vi "PPL_ActionVIOnCompile.vi"(8 "error in (no error)":errorcluster, 11 "Device Item Ref in":T1 format="%.0x") -> (0 "error out":errorcluster)   [LabVIEW 2019]
uses:
  <vilib>/NI VeriStand/Custom Device API/Custom Device Item Ref.ctl
  <vilib>/NI VeriStand/Custom Device Tools/Custom Device Utility Library/NI VeriStand - Search for Item by Name.vi
  <vilib>/NI VeriStand/Custom Device API/Set Item Property (Variant).vi
  <vilib>/NI VeriStand/Custom Device Tools/Custom Device Utility Library/Custom Device Utility Library.lvlib
  <vilib>/NI VeriStand/Custom Device API/Custom Device API.lvlib
  <vilib>/NI/NIVS Inline Async API/_Data Access System Explorer/Data Access System Explorer.lvlib
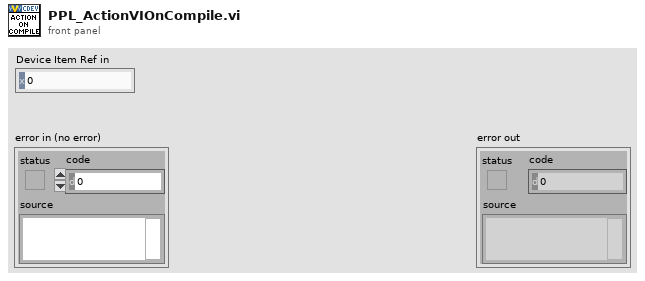
[diagram p1: front panel]
types:
  T1 = typedef "Custom Device API.lvlib/Custom Device Item Ref.ctl" = u64
  T2 = cluster{"Name":string, "Type":enum16{"Output/Write", "Input/Read", "Input/ReadWrite"}, "VS Refs":T1[]}
  T3 = enum16{"Output/Write", "Input/Read", "Input/ReadWrite"}
  T4 = typedef "Custom Device API.lvlib/Custom Device Item Info.ctl" = cluster{"Name":string, "Is Channel":bool, "GUID":string, "Is Waveform":bool}
  T5 = cluster{"Name":string, "Type":enum16{"Output/Write", "Input/Read", "Input/ReadWrite"}, "VS Refs":T1[]}[]
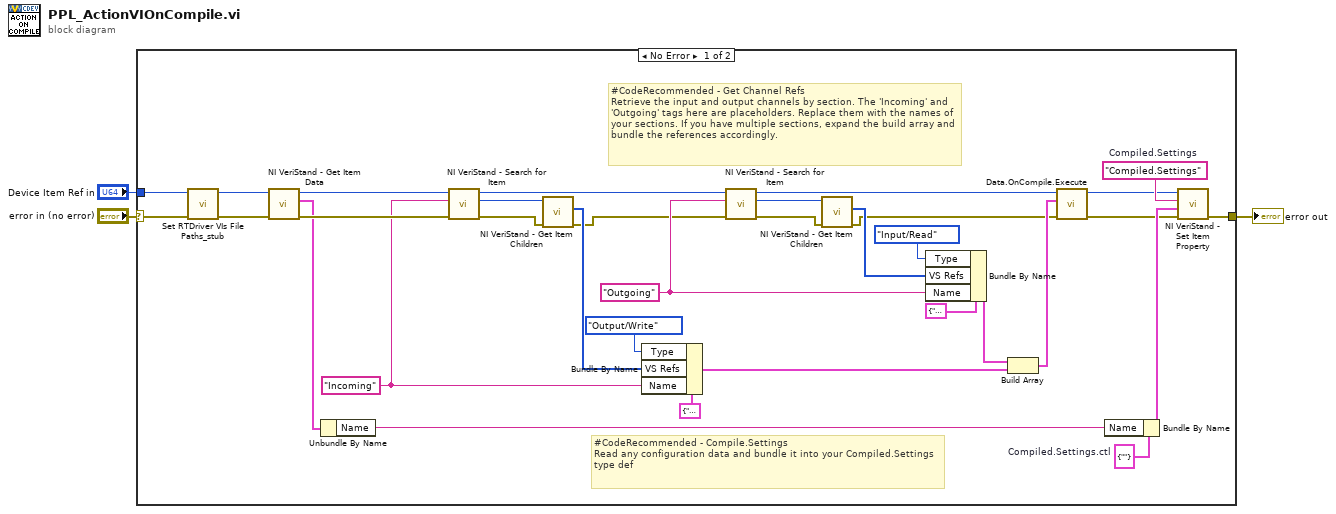
[diagram p0: block diagram]
diagram:
  n1 = case shown="No Error" "error in (no error)" {
    selector: "error in (no error)" -> [w4 w37]
    tunnel: [w30 w37] -> w2
    tunnel: "Device Item Ref in" -> [w7 _]
    frame No Error {
      w8 = cluster{"Name":string} {"Name"=""}  # Compiled.Settings.ctl
      w23 = "Outgoing" ("Item Name")
      w25 = "Incoming" ("Item Name")
      w32 = "Compiled.Settings"  # Compiled.Settings
      # "#CodeRecommended - Get Channel Refs\nRetrieve the input and output channels by section. The 'Incoming' and 'Outgoing' tags here are placeholders. Replace them with the names of your sections. If you have multiple sections, expand the build array and bundle the references accordingly."
      # "#CodeRecommended - Compile.Settings\nRead any configuration data and bundle it into your Compiled.Settings type def"
      n2 = call "Set RTDriver VIs File Paths_stub.vi"("error in (no error)"=w4, "Item Ref in"=w7) -> ("error out"=w5:errorcluster, "Item Ref out"=w6:T1)  [unwired: 8 in]
      n3 = call <vilib>:"NI VeriStand - Get Item Data.vi"("error in (no error)"=w5, "Item Ref in"=w6) -> ("error out"=w28:errorcluster, "Item Info"=w27:T4, "Item Ref out"=w29:T1)  [unwired: 6 in, 1 out]
      n4 = Unbundle By Name(w27) -> ("Name"=w26:string)
      n5 = call-poly <vilib>:"NI VeriStand - Search for Item.vi"("error in"=w28, "Item Name"=w25, "Section Ref in"=w29) -> ("error out"=w36:errorcluster, "Item Ref"=w35:T1, "Section Ref out"=w12:T1)  [unwired: 5 in, 1 out]
      n6 = call <vilib>:"NI VeriStand - Get Item Children.vi"("error in (no error)"=w36, "Item Ref in"=w35) -> ("error out"=w11:errorcluster, "Child Refs"=w24:T1[])  [unwired: 6 in, 2 out]
      n7 = Bundle By Name(cluster=T2 {"Name"="", "Type"=enum."Output/Write", "VS Refs"=[]} ("Group"), "Type"=T3."Output/Write", "VS Refs"=w24, "Name"=w25) -> (w15:T2)
      n8 = call-poly <vilib>:"NI VeriStand - Search for Item.vi"("error in"=w11, "Item Name"=w23, "Section Ref in"=w12) -> ("error out"=w33:errorcluster, "Item Ref"=w34:T1, "Section Ref out"=w13:T1)  [unwired: 5 in, 1 out]
      n9 = call <vilib>:"NI VeriStand - Get Item Children.vi"("error in (no error)"=w33, "Item Ref in"=w34) -> ("error out"=w14:errorcluster, "Child Refs"=w19:T1[])  [unwired: 6 in, 2 out]
      n10 = Bundle By Name(cluster=T2 {"Name"="", "Type"=enum."Output/Write", "VS Refs"=[]} ("Group"), "Type"=T3."Input/Read", "VS Refs"=w19, "Name"=w23) -> (w21:T2)
      n11 = Build Array(w21, w15) -> (w18:T5)
      n12 = call <vilib>:"Data.OnCompile.Execute.vi"("error in"=w14, "VS Ref Groups"=w18, "Custom Device Ref"=w13) -> ("error out"=w10:errorcluster, "Custom Device Ref"=w9:T1)  [unwired: 7 in]
      n13 = Bundle By Name(cluster=w8, "Name"=w26) -> (w31:cluster{"Name":string})
      n14 = call-poly <vilib>:"NI VeriStand - Set Item Property.vi"("error in (no error)"=w10, "Value"=w31, "Property Name"=w32, "Item Ref in"=w9) -> ("error out"=w30:errorcluster)  [unwired: 5 in, 2 out]
    }
    frame Error {
    }
  }
  "error out" <- w2
